vi "Format Image.vi"(1 "Picture Color Type":T1, 4 "Picture Index":i32=-1, 5 "Measurement System":T2=enum."Metric", 6 "error in (no error)":errorcluster, 7 "Width":dbl=-1.0, 8 "Scale Factor":dbl=1.0, 9 "Height":dbl=-1.0, 10 "Report Ref In":T3) -> (0 "error out":errorcluster, 3 "Report Ref Out":T3)   [LabVIEW 2026, in "XCel Report Engine.lvlib"]
uses:
  XCel Report Engine.lvlib
  Controls/Report Ref.ctl
  C:/Users/m.santucci/Documents/ChatGPT/LV_REPORT_ENGINE/LV/DotNet/XCelReportEngine.dll
  DotNet/XCelReportEngine.dll
  Controls/Measurement System.ctl
  Controls/Picture Color Type.ctl
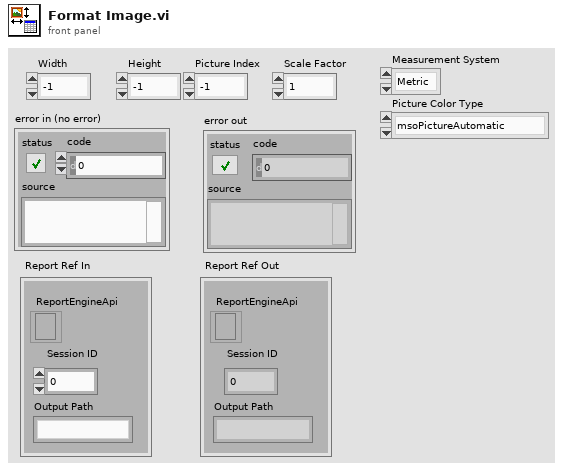
[diagram p1: front panel]
types:
  T1 = typedef "XCel Report Engine.lvlib/Picture Color Type.ctl" = enum32{"msoPictureAutomatic", "msoPictureMixed", "msoPictureGrayscale", "msoPictureBlack&White", "msoPictureWatermark"}
  T2 = typedef "XCel Report Engine.lvlib/Measurement System.ctl" = enum32{"US", "Metric"}
  T3 = typedef "XCel Report Engine.lvlib/Report Ref.ctl" = cluster{"Session ID":i32, "Output Path":string, "ReportEngineApi":refnum<k24>}
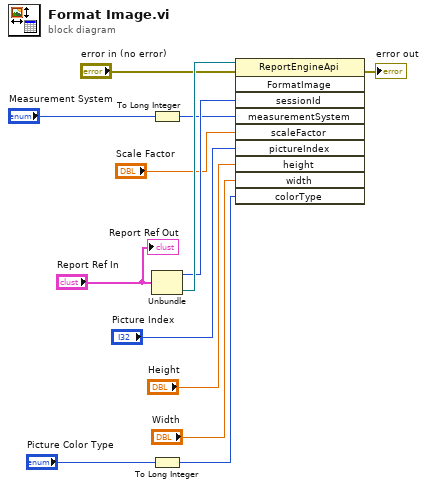
[diagram p0: block diagram]
diagram:
  n1 = To Long Integer(number="Measurement System") -> (32bit integer=w3:i32)
  n2 = Unbundle("Report Ref In") -> ("Session ID"=w9:i32, "ReportEngineApi"=w12:refnum<k24>)  [unwired: 1 out]
  n3 = To Long Integer(number="Picture Color Type") -> (32bit integer=w5:i32)
  n4 = invoke class="ReportEngineApi" method="FormatImage"(reference=w12, error in="error in (no error)", "sessionId"=w9, "measurementSystem"=w3, "scaleFactor"="Scale Factor", "pictureIndex"="Picture Index", "height"="Height", "width"="Width", "colorType"=w5) -> (error out=→"error out":errorcluster)  [unwired: 1 in, 9 out]
  "Report Ref Out" <- "Report Ref In"
